vi "list_box_filter.vi"() -> ()   [LabVIEW 2017]
panel:
  in  "Input selection subarry":string[][](array[string])=[["03/22/2019", "201", "1", "1"], ["03/22/2019", "201", "1", "2"], ["03/22/2019", "204", "2", "1"], ["03/22/2019", "204", "3", "2"], ["03/22/2018", "205", "4", ""], ["03/22/2018", "206", "5", ""], ["03/22/2018", "207", "7", ""], ["03/22/2018", "208", "7", ""]]
  out "BarWO Select Output Subarry":string[][](array[string])=[["03/22/2019", "201", "1", "1"], ["03/22/2019", "201", "1", "2"], ["03/22/2019", "204", "3", "2"]]
  out "BarSN":string[](array[string])=["201", "204", "All"]
  out "BarWO":string[](array[string])=["1", "2", "3", "4", "5", "7", "All"]
  out "WaferID Select Output Subarry":string[][](array[string])=[["03/22/2019", "201", "1", "1"], ["03/22/2019", "201", "1", "2"], ["03/22/2019", "204", "2", "1"], ["03/22/2019", "204", "3", "2"], ["03/22/2018", "205", "4", ""], ["03/22/2018", "206", "5", ""], ["03/22/2018", "207", "7", ""], ["03/22/2018", "208", "7", ""]]
  out "WaferID":string[](array[string])=["1", "2", "All"]
  in  "Test Date Selection":i32[](listbox)=[0]
  in  "Bar SN Selection":i32[](listbox)
  in  "Bar WO Selection":i32[](listbox)
  in  "Wafer ID Selection":i32[](listbox)=[2]
  # "This function accepts 2D array,  for each column it filters out the unique selection items. \nMake the selections, then update the rest of the selection box."
  # "Eempty strings have been removed. If choose all, it will include empty string selections"
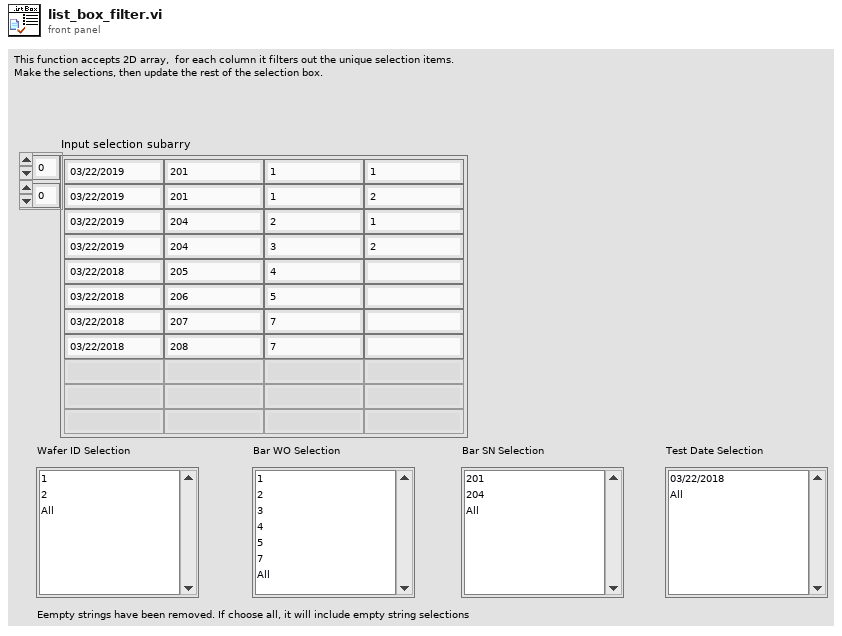
[diagram p1: front panel]
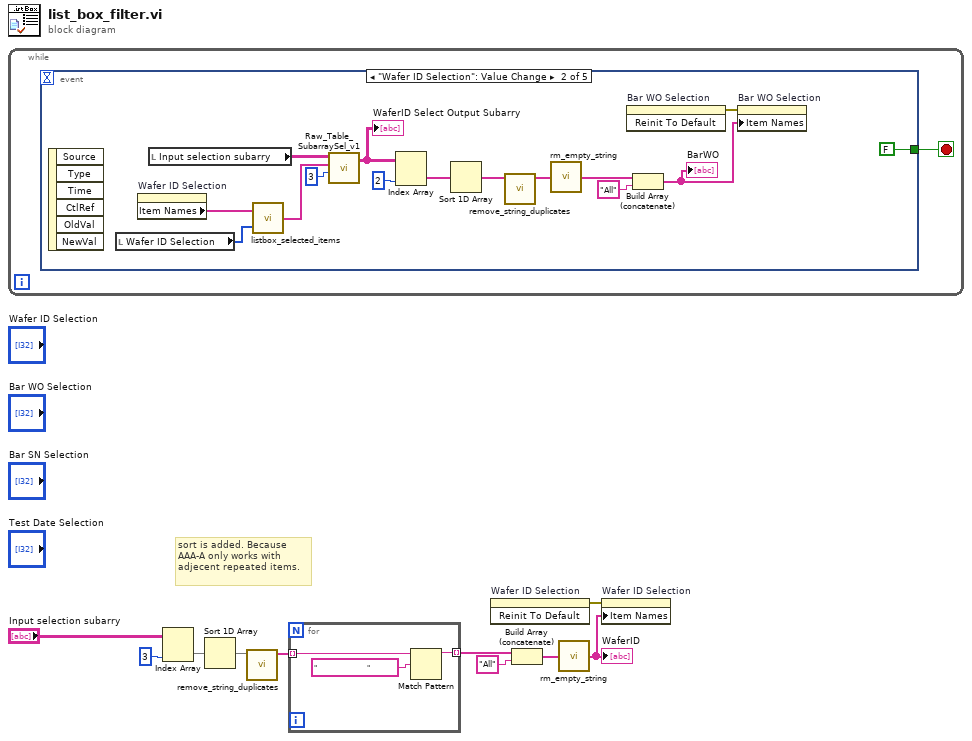
[diagram p0: block diagram]
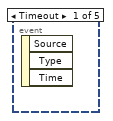
[diagram p2: hidden frame]
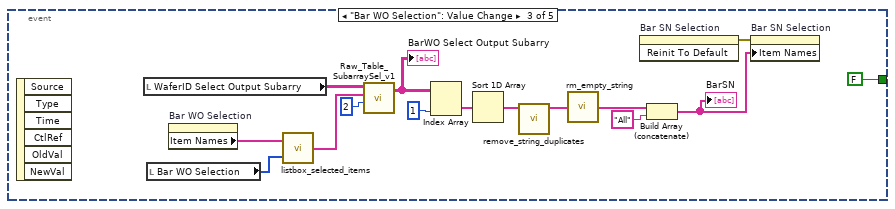
[diagram p3: hidden frame]
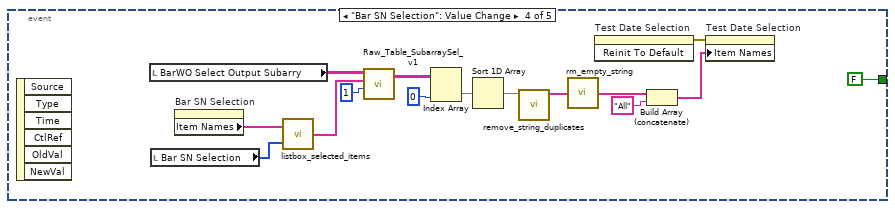
[diagram p4: hidden frame]
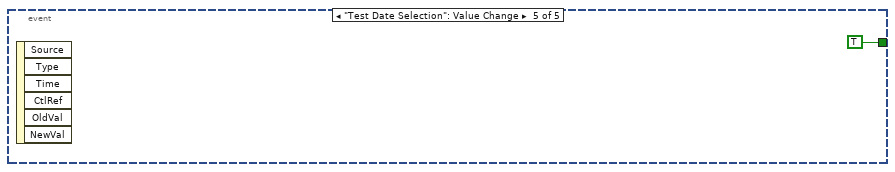
[diagram p5: hidden frame]
diagram:
  # "sort is added. Because AAA-A only works with adjecent repeated items."
  n1 = while {
    stop <- w11 stop-if-true
    n2 = event shown="[1] \"Wafer ID Selection\": Value Change" {
      selector: _ -> [_ _ _ _ _]
      dyn-events: _ -> [_ _ _ _ _]
      timeout: _ -> [_ _ _ _ _]
      tunnel: [_ FALSE ("stop") FALSE ("stop") FALSE ("stop") TRUE ("stop")] -> w11
      event Timeout {
        n3 = event-data() -> ()  [unwired: 1 in, 3 out]
      }
      event "Wafer ID Selection": Value Change {
        n4 = event-data() -> ()  [unwired: 1 in, 6 out]
        n5 = local read "Wafer ID Selection"() -> (w15:i32[])
        n6 = property on="Wafer ID Selection" class="LstBox (strict)"() -> ("Item Names"=w16:string[])  [unwired: 2 in, 2 out]
        n7 = local read "Input selection subarry"() -> (w26:string[][])
        n8 = call "listbox_selected_items.vi"("Selected item number"=w15, "All items"=w16) -> ("Selected items"=w14:string[])
        n9 = call "Raw_Table_SubarraySel_v1.vi"("Column Index"=3, "String to compare"=w14, "Raw Bar Table Data"=w26) -> ("Selected Output"=w23:string[][])  [unwired: 1 in, 1 out]
        "WaferID Select Output Subarry" <- w23
        n10 = Index Array(array=w23, index (col)=2 ("disabled index (col)")) -> (element=w13:string[])  [unwired: 1 in]
        n11 = Sort 1D Array(array=w13) -> (sorted array=w12:string[])
        n12 = call "remove_string_duplicates.vi"("In"=w12) -> ("Out"=w19:string[])  [unwired: 10 in]
        n13 = call "rm_empty_string.vi"("Array"=w19) -> ("String output"=w21:string[])
        n14 = invoke on="Bar WO Selection" class="LstBox (strict)" method="Reinit To Default"() -> (error out=w17:errorcluster)  [unwired: 3 in, 2 out]
        n15 = Build Array (concatenate)(w21, "All") -> (w18:string[])
        "BarWO" <- w18
        n16 = property on="Bar WO Selection" class="LstBox (strict)"(error in=w17, "Item Names"=w18) -> ()  [unwired: 1 in, 2 out]
      }
      event "Bar WO Selection": Value Change {
        n17 = event-data() -> ()  [unwired: 1 in, 6 out]
        n18 = local read "WaferID Select Output Subarry"() -> (w41:string[][])
        n19 = local read "Bar WO Selection"() -> (w30:i32[])
        n20 = property on="Bar WO Selection" class="LstBox (strict)"() -> ("Item Names"=w31:string[])  [unwired: 2 in, 2 out]
        n21 = call "listbox_selected_items.vi"("Selected item number"=w30, "All items"=w31) -> ("Selected items"=w29:string[])
        n22 = call "Raw_Table_SubarraySel_v1.vi"("Column Index"=2, "String to compare"=w29, "Raw Bar Table Data"=w41) -> ("Selected Output"=w39:string[][])  [unwired: 1 in, 1 out]
        "BarWO Select Output Subarry" <- w39
        n23 = Index Array(array=w39, index (col)=1 ("disabled index (col)")) -> (element=w28:string[])  [unwired: 1 in]
        n24 = Sort 1D Array(array=w28) -> (sorted array=w27:string[])
        n25 = call "remove_string_duplicates.vi"("In"=w27) -> ("Out"=w34:string[])  [unwired: 10 in]
        n26 = call "rm_empty_string.vi"("Array"=w34) -> ("String output"=w36:string[])
        n27 = invoke on="Bar SN Selection" class="LstBox (strict)" method="Reinit To Default"() -> (error out=w32:errorcluster)  [unwired: 3 in, 2 out]
        n28 = Build Array (concatenate)(w36, "All") -> (w33:string[])
        "BarSN" <- w33
        n29 = property on="Bar SN Selection" class="LstBox (strict)"(error in=w32, "Item Names"=w33) -> ()  [unwired: 1 in, 2 out]
      }
      event "Bar SN Selection": Value Change {
        n30 = event-data() -> ()  [unwired: 1 in, 6 out]
        n31 = local read "BarWO Select Output Subarry"() -> (w56:string[][])
        n32 = local read "Bar SN Selection"() -> (w45:i32[])
        n33 = property on="Bar SN Selection" class="LstBox (strict)"() -> ("Item Names"=w46:string[])  [unwired: 2 in, 2 out]
        n34 = call "listbox_selected_items.vi"("Selected item number"=w45, "All items"=w46) -> ("Selected items"=w44:string[])
        n35 = call "Raw_Table_SubarraySel_v1.vi"("Column Index"=1, "String to compare"=w44, "Raw Bar Table Data"=w56) -> ("Selected Output"=w54:string[][])  [unwired: 1 in, 1 out]
        n36 = Index Array(array=w54, index (col)=0 ("disabled index (col)")) -> (element=w43:string[])  [unwired: 1 in]
        n37 = Sort 1D Array(array=w43) -> (sorted array=w42:string[])
        n38 = call "remove_string_duplicates.vi"("In"=w42) -> ("Out"=w52:string[])  [unwired: 10 in]
        n39 = call "rm_empty_string.vi"("Array"=w52) -> ("String output"=w51:string[])
        n40 = invoke on="Test Date Selection" class="LstBox (strict)" method="Reinit To Default"() -> (error out=w47:errorcluster)  [unwired: 3 in, 2 out]
        n41 = Build Array (concatenate)(w51, "All") -> (w49:string[])
        n42 = property on="Test Date Selection" class="LstBox (strict)"(error in=w47, "Item Names"=w49) -> ()  [unwired: 1 in, 2 out]
      }
      event "Test Date Selection": Value Change {
        n43 = event-data() -> ()  [unwired: 1 in, 6 out]
      }
    }
  }
  n44 = Index Array(array="Input selection subarry", index (col)=3 ("disabled index (col)")) -> (element=w3:string[])  [unwired: 1 in]
  n45 = Sort 1D Array(array=w3) -> (sorted array=w2:string[])
  n46 = call "remove_string_duplicates.vi"("In"=w2) -> ("Out"=w7:string[])  [unwired: 10 in]
  n47 = for {
    tunnel: w7 -> [w60] mode=indexing
    tunnel: [w58] -> w6 mode=indexing
    n48 = Match Pattern(string=w60, regular expression="                         ") -> (before substring=w58:string)  [unwired: 1 in, 3 out]
  }
  n49 = invoke on="Wafer ID Selection" class="LstBox (strict)" method="Reinit To Default"() -> (error out=w4:errorcluster)  [unwired: 3 in, 2 out]
  n50 = Build Array (concatenate)(w6, "All") -> (w5:string[])
  n51 = call "rm_empty_string.vi"("Array"=w5) -> ("String output"=w1:string[])
  "WaferID" <- w1
  n52 = property on="Wafer ID Selection" class="LstBox (strict)"(error in=w4, "Item Names"=w1) -> ()  [unwired: 1 in, 2 out]
